vi "Practica6.1_Clusters.vi"() -> ()   [LabVIEW 2022 SP3]
panel:
  out "Salida sin nombre":T1
  out "Salida por nombre":T1
  out "Negación de activación":bool
  in  "Entrada de datos":T1 {"Variación de entrada" scale=0.0..10.0; "Intensidad" scale=0.0..50.0}
  # "Anahí Montserrat Vázquez Padilla \nPráctica 06: Clusters\n14/02/2024"
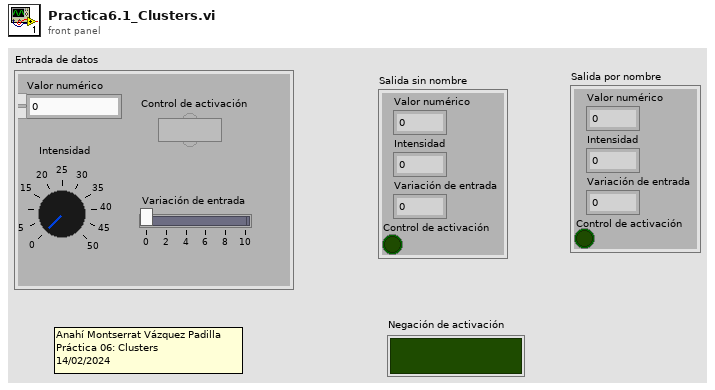
[diagram p1: front panel]
types:
  T1 = cluster{"Valor numérico":dbl, "Intensidad":dbl, "Variación de entrada":dbl, "Control de activación":bool}
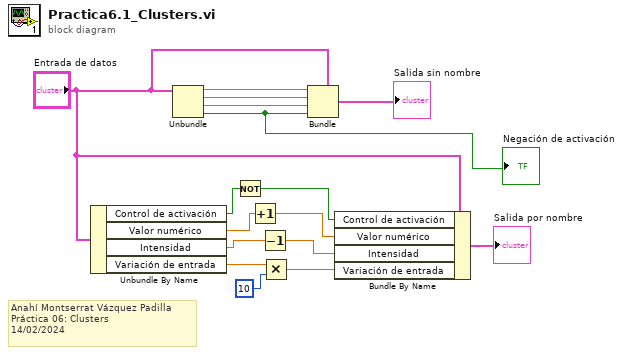
[diagram p0: block diagram]
diagram:
  # "Anahí Montserrat Vázquez Padilla \nPráctica 06: Clusters\n14/02/2024"
  n1 = Unbundle By Name "Unbundle By Name"("Entrada de datos") -> ("Control de activación"=w10:bool, "Valor numérico"=w8:dbl, "Intensidad"=w6:dbl, "Variación de entrada"=w4:dbl)
  n2 = Unbundle "Unbundle"("Entrada de datos") -> ("Valor numérico"=w16:dbl, "Intensidad"=w12:dbl, "Variación de entrada"=w15:dbl, "Control de activación"=w11:bool)
  "Negación de activación" <- w11
  n3 = Not(x=w10) -> (.not. x?=w9:bool)
  n4 = Increment(x=w8) -> (x+1=w7:dbl)
  n5 = Decrement(x=w6) -> (x-1=w5:dbl)
  n6 = Multiply(x=w4, y=10) -> (x*y=w3:dbl)
  n7 = Bundle "Bundle"(cluster="Entrada de datos", "Valor numérico"=w16, "Intensidad"=w12, "Variación de entrada"=w15, "Control de activación"=w11) -> (→"Salida sin nombre":T1)
  n8 = Bundle By Name "Bundle By Name"(cluster="Entrada de datos", "Control de activación"=w9, "Valor numérico"=w7, "Intensidad"=w5, "Variación de entrada"=w3) -> (→"Salida por nombre":T1)
